vi "U32 array to Hex.vi"(11 "Array":u32[](array[numeric])) -> (3 "Hex string":string)   [LabVIEW 2020, in "wamplv.lvlib" / "Utils.lvclass"]
uses:
  Utils.lvclass
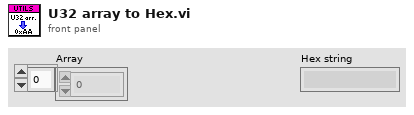
[diagram p1: front panel]
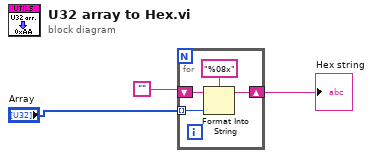
[diagram p0: block diagram]
diagram:
  n1 = for {
    tunnel: "Array" -> [w7] mode=indexing
    shift-right: [w6] -> w1
    shift-left: "" -> [w5]
    n2 = Format Into String(format string="%08x", initial string=w5, w7) -> (resulting string=w6:string)  [unwired: 1 in, 1 out]
  }
  "Hex string" <- w1
